vi "test.vi"() -> ()   [LabVIEW 2013]
panel:
  out "output array":i32[](array[numeric])
  in  "Boolean":bool
  in  "stop":bool
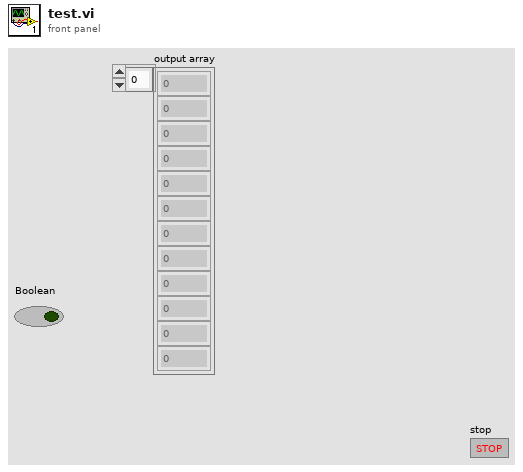
[diagram p1: front panel]
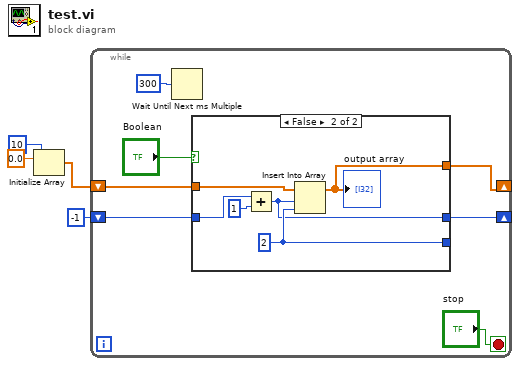
[diagram p0: block diagram]
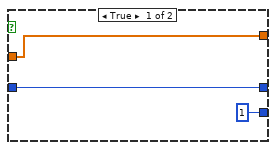
[diagram p2: hidden frame]
diagram:
  n1 = Initialize Array(0.0 ("element"), 10 ("dimension size")) -> (w3:dbl[])
  n2 = while {
    shift-right: [w7] -> _
    shift-left: -1 -> [w8]
    shift-right: [w5] -> _
    shift-left: w3 -> [w6]
    stop <- "stop" stop-if-true
    n3 = Wait Until Next ms Multiple(millisecond multiple=u32 300) -> ()  [unwired: 1 out]
    n4 = case shown="False" "Boolean" {
      tunnel: [1 w20] -> _
      tunnel: w8 -> [w13 w19]
      tunnel: [w13 w17] -> w7
      tunnel: w6 -> [w12 w16]
      tunnel: [w12 w15] -> w5
      frame True {
      }
      frame False {
        w20 = 2
        n5 = Add(x=w19, y=1) -> (x+y=w17:i32)
        n6 = Insert Into Array(array=w16, index=w17, new element=w20) -> (w15:dbl[])
        "output array" <- w15
      }
    }
  }
